vi "Test Column Letter To Number.vi"(11 "Test Case In":refnum<class "Test Open Xml.lvclass">) -> (0 "error out":errorcluster, 3 "Test Case Out":refnum<class "Test Open Xml.lvclass">)   [LabVIEW 2021, in "Test Open Xml.lvclass"]
uses:
  Test Open Xml.lvclass
  C:/Program Files/National Instruments/LabVIEW 2025/vi.lib/Astemes/LUnit/Test Case.lvclass
  <vilib>/Astemes/LUnit/Test Case.lvclass/Test Case.ctl
  Source/Open Xml.lvlib
  <vilib>/Astemes/LUnit/Test Case.lvclass
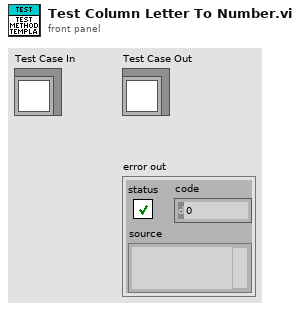
[diagram p1: front panel]
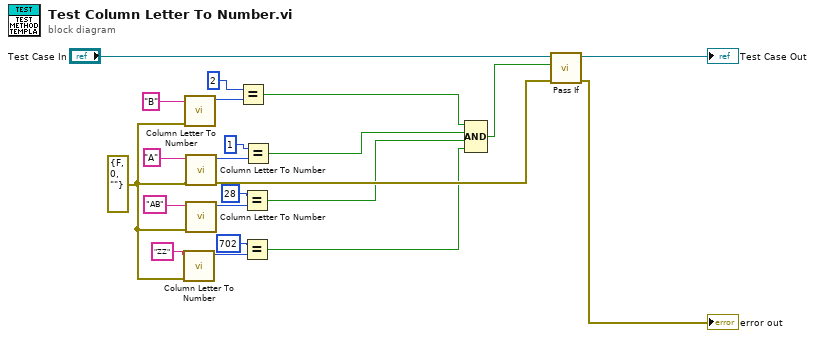
[diagram p0: block diagram]
diagram:
  w10 = errorcluster {"status"=FALSE, "code"=0, "source"=""} ("error in")
  n1 = call "Column Letter To Number.vi"("error in"=w10, "Letter"="ZZ") -> ("Number"=w7:i32)  [unwired: 8 in, 1 out]
  n2 = call "Column Letter To Number.vi"("error in"=w10, "Letter"="B") -> ("Number"=w9:i32)  [unwired: 8 in, 1 out]
  n3 = call "Column Letter To Number.vi"("error in"=w10, "Letter"="A") -> ("error out"=w16:errorcluster, "Number"=w18:i32)  [unwired: 8 in]
  n4 = call "Column Letter To Number.vi"("error in"=w10, "Letter"="AB") -> ("Number"=w14:i32)  [unwired: 8 in, 1 out]
  n5 = Equal?(x=2, y=w9) -> (x = y?=w5:bool)
  n6 = Equal?(x=28, y=w14) -> (x = y?=w3:bool)
  n7 = Equal?(x=702, y=w7) -> (x = y?=w2:bool)
  n8 = Equal?(x=1, y=w18) -> (x = y?=w4:bool)
  n9 = Compound Arithmetic op=AND(w5, w4, w3, w2) -> (w1:bool)
  n10 = call <vilib>:"Pass If.vi"("error in (no error)"=w16, "Pass?"=w1, "LUnit Test Case In"="Test Case In") -> ("error out"=→"error out":errorcluster, "LUnit Test Case Out"=→"Test Case Out":refnum<class "Test Open Xml.lvclass">)  [unwired: 7 in]
